vi "Set SN.vi"(8 "error in (no error)":errorcluster caption="entrée d'erreur (pas d'erreur)", 10 "SN":string, 11 "Creation_SN (Virtual) en entrée":refnum<class "Creation_SN (Virtual).lvclass">) -> (0 "error out":errorcluster caption="sortie d'erreur", 3 "Creation_SN (Virtual) en sortie":refnum<class "Creation_SN (Virtual).lvclass">)   [LabVIEW 2020, in "Library Instrument & Equipement.lvlib" / "Library Creation_SN.lvlib" / "Creation_SN (Virtual).lvclass"]
uses:
  Creation_SN (Virtual).lvclass
  Creation_SN (Virtual).lvclass/Creation_SN (Virtual).ctl
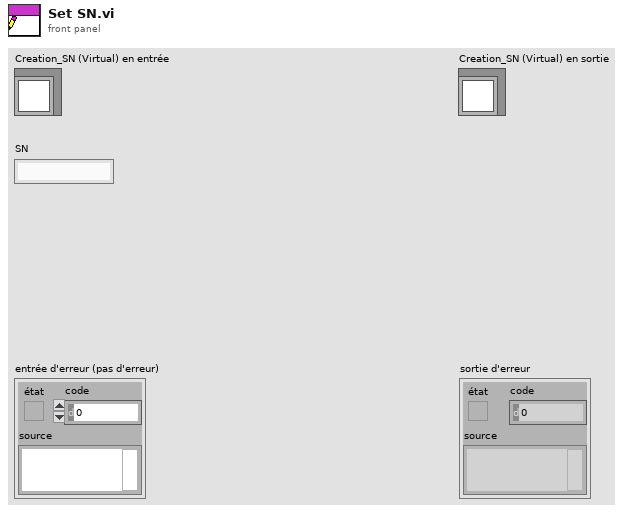
[diagram p1: front panel]
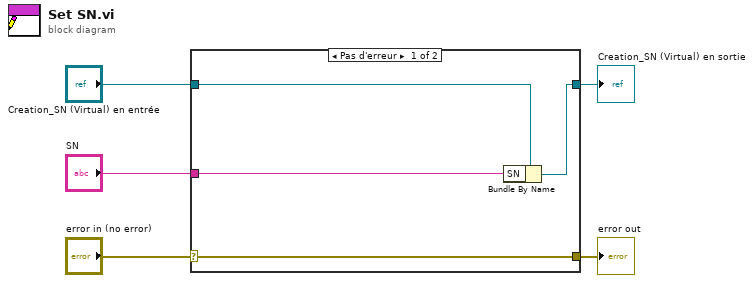
[diagram p0: block diagram]
diagram:
  n1 = case shown="Pas d'erreur" "error in (no error)" {
    selector: "error in (no error)" -> [w9 w10]
    tunnel: [w9 w10] -> w4
    tunnel: [w7 w11] -> w2
    tunnel: "Creation_SN (Virtual) en entrée" -> [w8 w11]
    tunnel: "SN" -> [w6 _]
    frame No Error {
      n2 = Bundle By Name(cluster=w8, "SN"=w6) -> (w7:refnum<class "Creation_SN (Virtual).lvclass">)
    }
    frame Error {
    }
  }
  "error out" <- w4
  "Creation_SN (Virtual) en sortie" <- w2
